vi "CSM - Convert Data to HexStr.vi"(2 "Variant":variant) -> (7 "HEX String (0-9,A-F)":string)   [LabVIEW 2017, in "Communicable State Machine.lvlib"]
doc: "### CSM - Convert Data to HexStr.vi\n\nConverts any LabVIEW data type to a HEXSTR format parameter string.\n\n> [!NOTE] CSM HEXSTR Format Parameters\n> To pass any data type in CSM parameters, CSM provides a default parameter format called HEXSTR for passing any data type.\n> HEXSTR: Converts any LabVIEW data type to a variant, then represents this variant's memory format as a hexadecimal string for passing in CSM parameters.\n> HEXSTR can be safely used as a state parameter without disrupting the parsing of CSM message strings.\n\n\n-- <b>Controls</b> --\n- <b>Variant</b>: LabVIEW data, supports any data type through variants\n\n-- <b>Indicators</b> --\n- <b>HEXSTR</b>: CSM HEXSTR format parameter"
uses:
  Communicable State Machine.lvlib
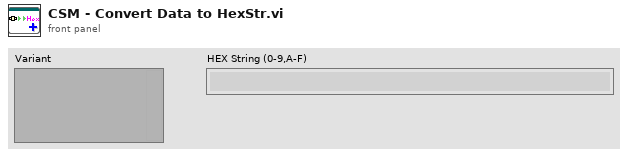
[diagram p1: front panel]
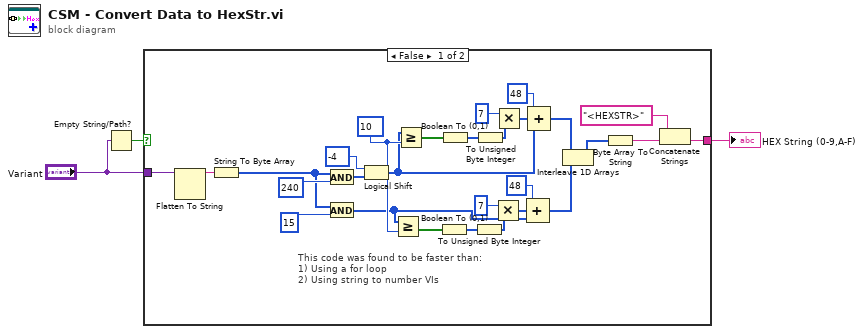
[diagram p0: block diagram]
diagram:
  n1 = Empty String/Path?(string/path="Variant") -> (empty?=w1:bool)
  n2 = case shown="False" w1 {
    tunnel: [w5 _] -> w3
    tunnel: "Variant" -> [w6 _]
    frame False {
      w26 = u8 10
      # "This code was found to be faster than:\n1) Using a for loop\n2) Using string to number VIs"
      n3 = Flatten To String(anything=w6) -> (data string=w31:string)  [unwired: 3 in, 2 out]
      n4 = String To Byte Array(string=w31) -> (unsigned byte array=w7:u8[])
      n5 = And(x=w7, y=u8 240) -> (x .and. y?=w28:u8[])
      n6 = And(x=w7, y=u8 15) -> (x .and. y?=w10:u8[])
      n7 = Logical Shift(y=i8 -4, x=w28) -> (x << y=w19:u8[])
      n8 = Greater Or Equal?(x=w10, y=w26) -> (x >= y?=w11:bool[])
      n9 = Greater Or Equal?(x=w19, y=w26) -> (x >= y?=w20:bool[])
      n10 = Boolean To (0,1)(Boolean=w11) -> (0, 1=w13:i16[])
      n11 = Boolean To (0,1)(Boolean=w20) -> (0, 1=w25:i16[])
      n12 = To Unsigned Byte Integer(number=w13) -> (unsigned 8bit integer=w14:u8[])
      n13 = To Unsigned Byte Integer(number=w25) -> (unsigned 8bit integer=w24:u8[])
      n14 = Multiply(x=u8 7, y=w14) -> (x*y=w16:u8[])
      n15 = Multiply(x=u8 7, y=w24) -> (x*y=w22:u8[])
      n16 = Compound Arithmetic op=ADD(u8 48, w16, w10) -> (w9:u8[])
      n17 = Compound Arithmetic op=ADD(u8 48, w22, w19) -> (w18:u8[])
      n18 = Interleave 1D Arrays(w18, w9) -> (w17:u8[])
      n19 = Byte Array To String(unsigned byte array=w17) -> (string=w8:string)
      n20 = Concatenate Strings("<HEXSTR>" ("string"), w8) -> (w5:string)
    }
    frame True {
    }
  }
  "HEX String (0-9,A-F)" <- w3
